vi "reflect.vi"(10 "xmax":dbl[](array[numeric]), 11 "centroid":dbl[](array[numeric])) -> (3 "xr":dbl[](array[numeric]))   [LabVIEW 2015]
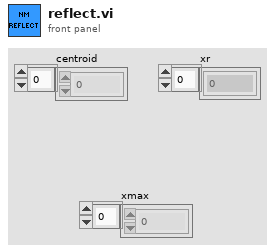
[diagram p1: front panel]
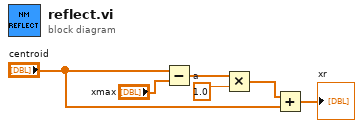
[diagram p0: block diagram]
diagram:
  w3 = 1.0  # a
  n1 = Subtract(x="centroid", y="xmax") -> (x-y=w2:dbl[])
  n2 = Multiply(x=w2, y=w3) -> (x*y=w4:dbl[])
  n3 = Add(x=w4, y="centroid") -> (x+y=→"xr":dbl[])
